vi "DAQWhichDevice.vi"(6 "error in":errorcluster caption="entrée d'erreur") -> (0 "error out":errorcluster caption="sortie d'erreur", 1 "AI.VoiesPhysiques":tag[](array[tag]), 2 "sourceTrig":tag, 3 "Message":string, 4 "DigitalInputFinAcq":tag, 5 "OK?":bool, 8 "Nom de périphérique DAQmx classique":tag)   [LabVIEW 2017]
uses:
  <resource>/objmgr/daqmx.rc
panel:
  out "AI.PhysicalChans":tag[](array[tag])
  out "error out 5":errorcluster
  out "résultat":i16
  out "0, 1":i16
  out "error out 4":errorcluster caption="sortie d'erreur"
  out "error out 3":errorcluster caption="sortie d'erreur"
  out "error out 2":errorcluster caption="sortie d'erreur"
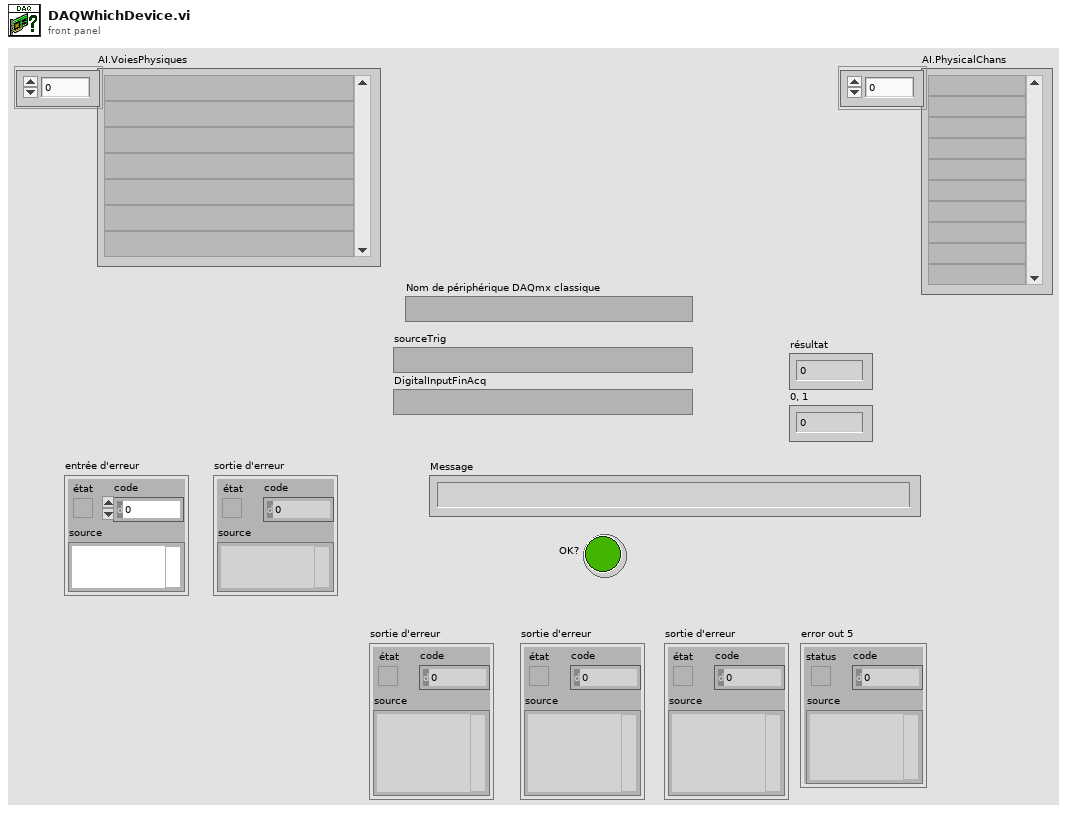
[diagram p1: front panel]
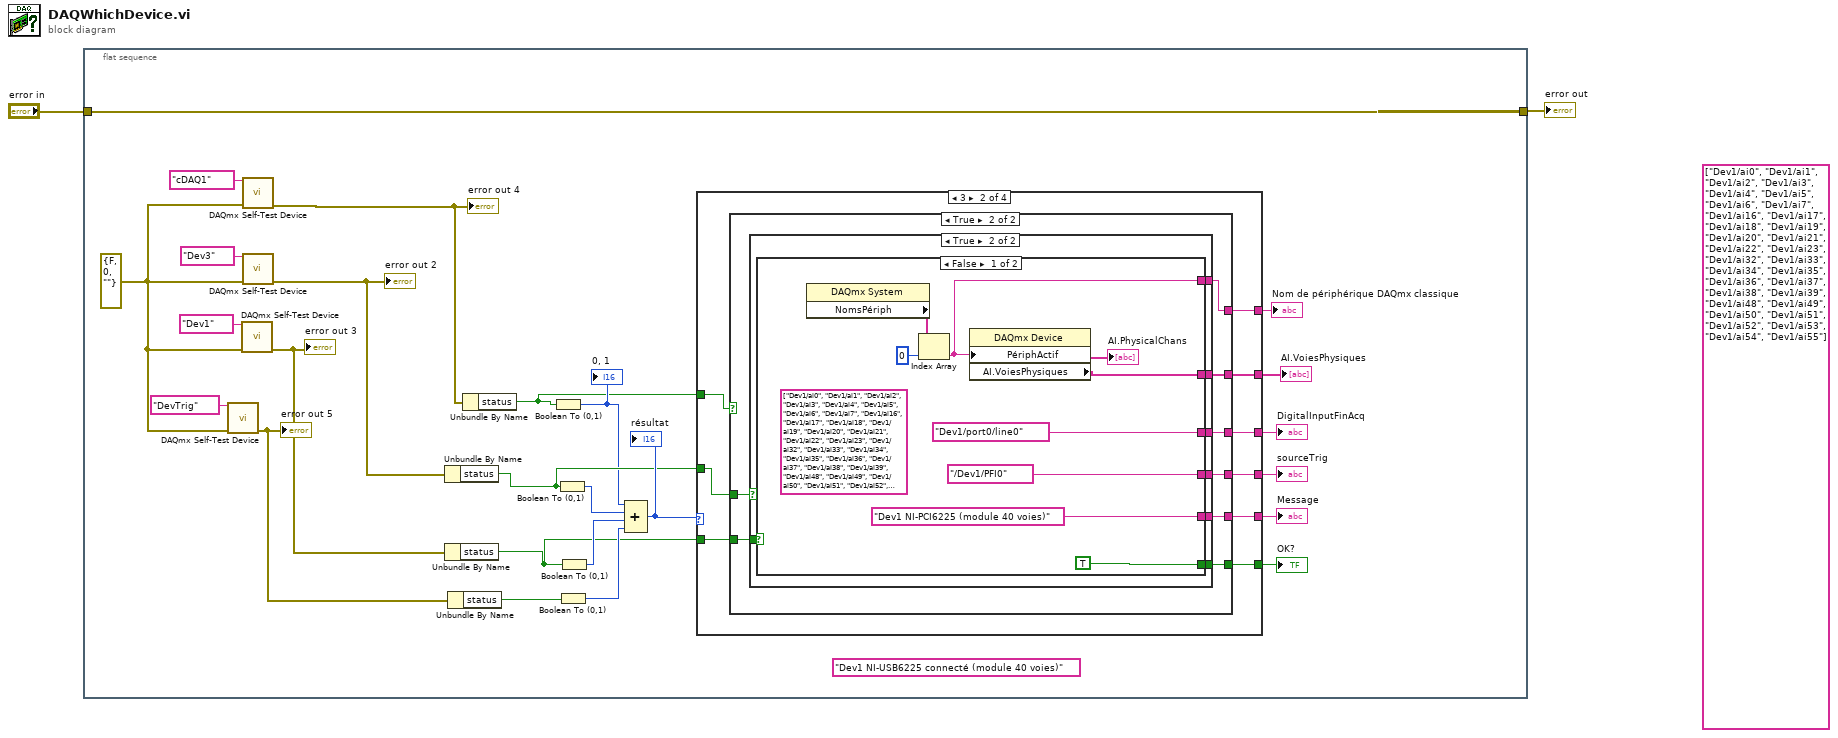
[diagram p0: block diagram]
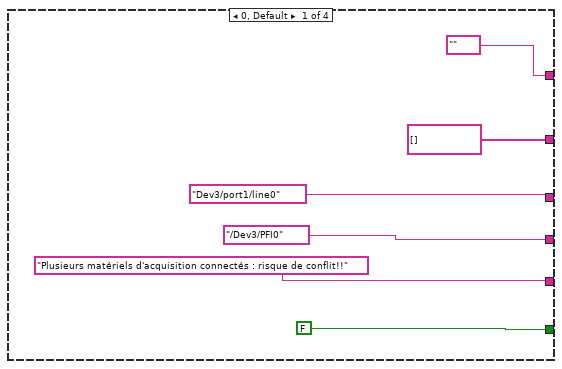
[diagram p2: hidden frame]
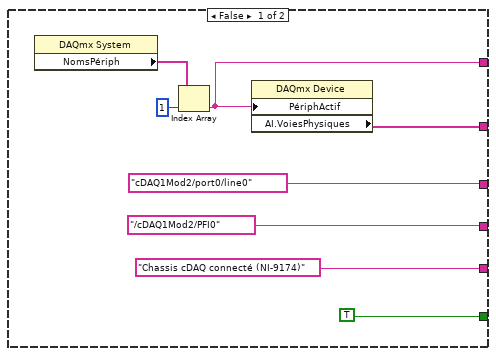
[diagram p3: hidden frame]
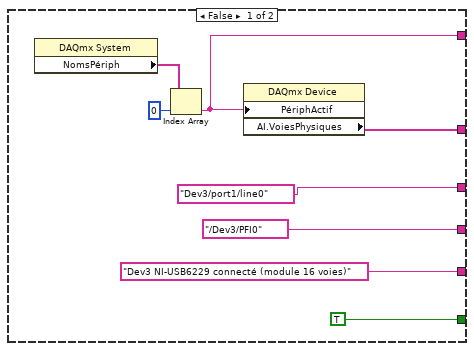
[diagram p4: hidden frame]
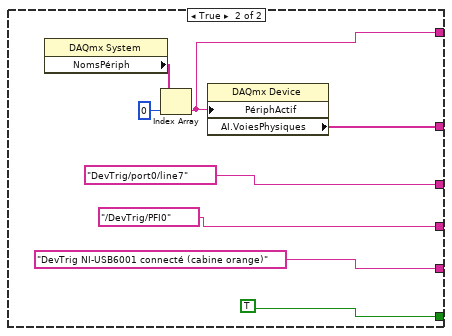
[diagram p5: hidden frame]
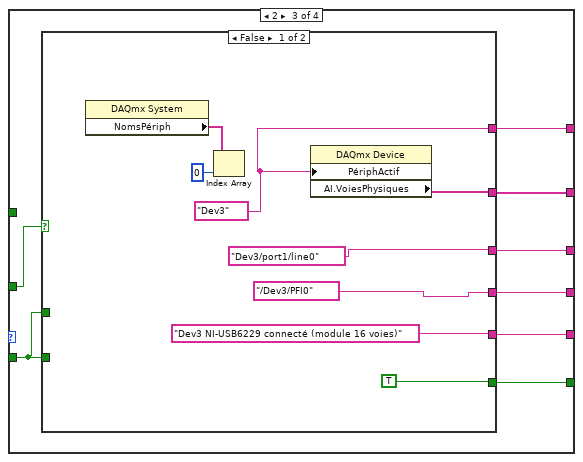
[diagram p6: hidden frame]
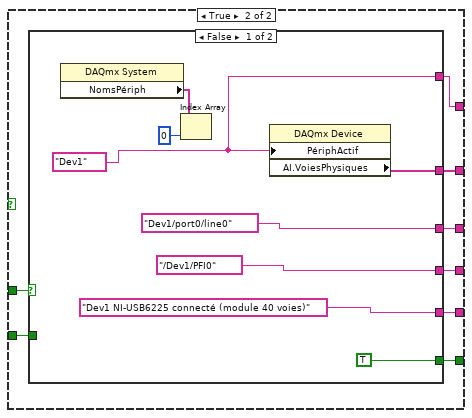
[diagram p7: hidden frame]
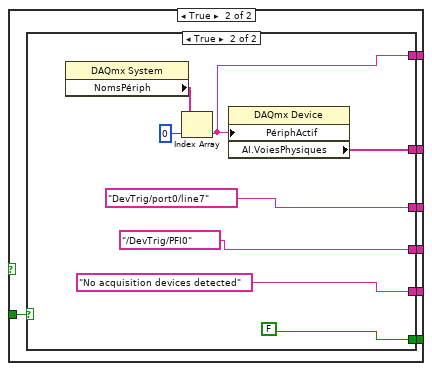
[diagram p8: hidden frame]
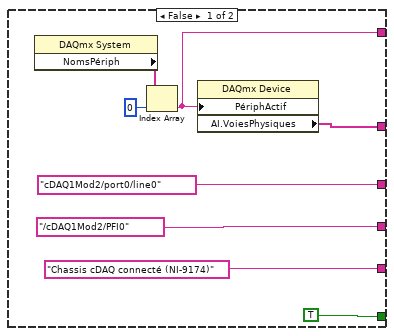
[diagram p9: hidden frame]
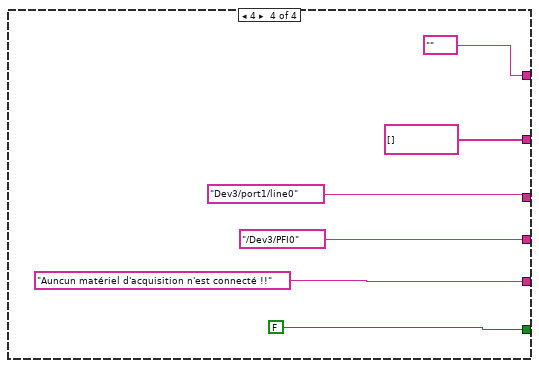
[diagram p10: hidden frame]
diagram:
  (unwired) tag[] ["Dev1/ai0", "Dev1/ai1", "Dev1/ai2", "Dev1/ai3", "Dev1/ai4", "Dev1/ai5", "Dev1/ai6", "Dev1/ai7", "Dev1/ai16", "Dev1/ai17", "Dev1/ai18", "Dev1/ai19", "Dev1/ai20", "Dev1/ai21", "Dev1/ai22", "Dev1/ai23", "Dev1/ai32", "Dev1/ai33", "Dev1/ai34", "Dev1/ai35", "Dev1/ai36", "Dev1/ai37", "Dev1/ai38", "Dev1/ai39", "Dev1/ai48", "Dev1/ai49", "Dev1/ai50", "Dev1/ai51", "Dev1/ai52", "Dev1/ai53", "Dev1/ai54", "Dev1/ai55"] ("AI.VoiesPhysiques 2")
  n1 = flat-sequence {
    tunnel: "error in" -> [w15]
    tunnel: [w15] -> w1
    frame #0 {
      (unwired) "Dev1 NI-USB6225 connecté (module 40 voies)"
      w7 = errorcluster {"status"=FALSE, "code"=0, "source"=""} ("error in")
      n2 = call <vilib>:"DAQmx Self-Test Device.vi"("device in"=tag "DevTrig", "error in"=w7) -> ("error out"=w5:errorcluster)  [unwired: 13 in]
      "error out 5" <- w5
      n3 = call <vilib>:"DAQmx Self-Test Device.vi"("device in"=tag "Dev1", "error in"=w7) -> ("error out"=w24:errorcluster)  [unwired: 13 in]
      "error out 3" <- w24
      n4 = call <vilib>:"DAQmx Self-Test Device.vi"("device in"=tag "cDAQ1", "error in"=w7) -> ("error out"=w13:errorcluster)  [unwired: 13 in]
      "error out 4" <- w13
      n5 = call <vilib>:"DAQmx Self-Test Device.vi"("device in"=tag "Dev3", "error in"=w7) -> ("error out"=w25:errorcluster)  [unwired: 13 in]
      "error out 2" <- w25
      n6 = Unbundle By Name(w25) -> ("status"=w17:bool)
      n7 = Unbundle By Name(w24) -> ("status"=w3:bool)
      n8 = Unbundle By Name(w5) -> ("status"=w6:bool)
      n9 = Unbundle By Name(w13) -> ("status"=w11:bool)
      n10 = Boolean To (0,1)(Boolean=w11) -> (0, 1=w12:i16)
      "0, 1" <- w12
      n11 = Boolean To (0,1)(Boolean=w17) -> (0, 1=w23:i16)
      n12 = Boolean To (0,1)(Boolean=w6) -> (0, 1=w4:i16)
      n13 = Boolean To (0,1)(Boolean=w3) -> (0, 1=w22:i16)
      n14 = Compound Arithmetic op=ADD(w12, w23, w22, w4) -> (w21:i16)
      "résultat" <- w21
      n15 = case shown="3" w21 {
        tunnel: ["Plusieurs matériels d'acquisition connectés : risque de conflit!!" w41 w97 "Auncun matériel d'acquisition n'est connecté !!"] -> w20
        tunnel: w17 -> [_ w42 w91 _]
        tunnel: [FALSE ("OK?") w40 w96 FALSE ("OK?")] -> w19
        tunnel: [tag "/Dev3/PFI0" ("source") w39 w95 tag "/Dev3/PFI0" ("source")] -> w18
        tunnel: [tag "Dev3/port1/line0" ("lines") w38 w94 tag "Dev3/port1/line0" ("lines")] -> w16
        tunnel: w11 -> [_ w37 _ _]
        tunnel: [tag[] [] ("AI.VoiesPhysiques") w36 w93 tag[] [] ("AI.VoiesPhysiques")] -> w10
        tunnel: [tag "" w35 w92 tag ""] -> w9
        tunnel: w3 -> [_ w34 w90 _]
        frame 0, Default {
        }
        frame 3 {
          n16 = case shown="True" w37 {
            tunnel: w42 -> [_ w58]
            tunnel: ["Chassis cDAQ connecté (NI-9174)" w57] -> w41
            tunnel: [TRUE ("OK?") w56] -> w40
            tunnel: [tag "/cDAQ1Mod2/PFI0" ("source") w55] -> w39
            tunnel: [tag "cDAQ1Mod2/port0/line0" ("lines") w54] -> w38
            tunnel: [w44 w53] -> w36
            tunnel: [w43 w52] -> w35
            tunnel: w34 -> [_ w51]
            frame False {
              n17 = property class="DAQmx System"() -> ("NomsPériph"=w45:tag[])  [unwired: 2 in, 2 out]
              n18 = Index Array(array=w45, index=1 ("indice")) -> (element=w43:tag)
              n19 = property class="DAQmx Device"("PériphActif"=w43) -> ("AI.VoiesPhysiques"=w44:tag[])  [unwired: 2 in, 2 out]
            }
            frame True {
              n20 = case shown="True" w58 {
                tunnel: ["Dev3 NI-USB6229 connecté (module 16 voies)" w73] -> w57
                tunnel: [TRUE ("OK?") w72] -> w56
                tunnel: [tag "/Dev3/PFI0" ("source") w71] -> w55
                tunnel: [tag "Dev3/port1/line0" ("lines") w70] -> w54
                tunnel: [w60 w67] -> w53
                tunnel: [w59 w69] -> w52
                tunnel: w51 -> [_ w68]
                frame False {
                  n21 = property class="DAQmx System"() -> ("NomsPériph"=w62:tag[])  [unwired: 2 in, 2 out]
                  n22 = Index Array(array=w62, index=0 ("indice")) -> (element=w59:tag)
                  n23 = property class="DAQmx Device"("PériphActif"=w59) -> ("AI.VoiesPhysiques"=w60:tag[])  [unwired: 2 in, 2 out]
                }
                frame True {
                  n24 = case shown="False" w68 {
                    tunnel: ["Dev1 NI-PCI6225 (module 40 voies)" "DevTrig NI-USB6001 connecté (cabine orange)"] -> w73
                    tunnel: [TRUE ("OK?") TRUE ("OK?")] -> w72
                    tunnel: [tag "/Dev1/PFI0" ("source") tag "/DevTrig/PFI0" ("source")] -> w71
                    tunnel: [tag "Dev1/port0/line0" ("lines") tag "DevTrig/port0/line7" ("lines")] -> w70
                    tunnel: [w74 w82] -> w67
                    tunnel: [w75 w87] -> w69
                    frame False {
                      (unwired) tag[] ["Dev1/ai0", "Dev1/ai1", "Dev1/ai2", "Dev1/ai3", "Dev1/ai4", "Dev1/ai5", "Dev1/ai6", "Dev1/ai7", "Dev1/ai16", "Dev1/ai17", "Dev1/ai18", "Dev1/ai19", "Dev1/ai20", "Dev1/ai21", "Dev1/ai22", "Dev1/ai23", "Dev1/ai32", "Dev1/ai33", "Dev1/ai34", "Dev1/ai35", "Dev1/ai36", "Dev1/ai37", "Dev1/ai38", "Dev1/ai39", "Dev1/ai48", "Dev1/ai49", "Dev1/ai50", "Dev1/ai51", "Dev1/ai52", "Dev1/ai53", "Dev1/ai54", "Dev1/ai55"] ("AI.VoiesPhysiques 2")
                      n25 = property class="DAQmx System"() -> ("NomsPériph"=w77:tag[])  [unwired: 2 in, 2 out]
                      n26 = Index Array(array=w77, index=0 ("indice")) -> (element=w75:tag)
                      n27 = property class="DAQmx Device"("PériphActif"=w75) -> ("AI.VoiesPhysiques"=w74:tag[])  [unwired: 2 in, 2 out]
                      "AI.PhysicalChans" <- w74
                    }
                    frame True {
                      n28 = property class="DAQmx System"() -> ("NomsPériph"=w89:tag[])  [unwired: 2 in, 2 out]
                      n29 = Index Array(array=w89, index=0 ("indice")) -> (element=w87:tag)
                      n30 = property class="DAQmx Device"("PériphActif"=w87) -> ("AI.VoiesPhysiques"=w82:tag[])  [unwired: 2 in, 2 out]
                    }
                  }
                }
              }
            }
          }
        }
        frame 2 {
          n31 = case shown="False" w91 {
            tunnel: w90 -> [_ w113]
            tunnel: ["Dev3 NI-USB6229 connecté (module 16 voies)" w112] -> w97
            tunnel: [TRUE ("OK?") w111] -> w96
            tunnel: [tag "/Dev3/PFI0" ("source") w110] -> w95
            tunnel: [tag "Dev3/port1/line0" ("lines") w109] -> w94
            tunnel: [w99 w108] -> w93
            tunnel: [w98 w107] -> w92
            tunnel: w90 -> [_ w106]
            frame False {
              w98 = tag "Dev3" ("device in")
              n32 = property class="DAQmx System"() -> ("NomsPériph"=w105:tag[])  [unwired: 2 in, 2 out]
              n33 = Index Array(array=w105, index=0 ("indice")) -> ()  [unwired: 1 out]
              n34 = property class="DAQmx Device"("PériphActif"=w98) -> ("AI.VoiesPhysiques"=w99:tag[])  [unwired: 2 in, 2 out]
            }
            frame True {
              n35 = case shown="False" w113 {
                tunnel: ["Dev1 NI-USB6225 connecté (module 40 voies)" w128] -> w112
                tunnel: [TRUE ("OK?") w127] -> w111
                tunnel: [tag "/Dev1/PFI0" ("source") w126] -> w110
                tunnel: [tag "Dev1/port0/line0" ("lines") w125] -> w109
                tunnel: [w118 w124] -> w108
                tunnel: [w114 w123] -> w107
                tunnel: w106 -> [_ w122]
                frame False {
                  w114 = tag "Dev1" ("Nom de périphérique DAQmx classique 2")
                  n36 = property class="DAQmx System"() -> ("NomsPériph"=w120:tag[])  [unwired: 2 in, 2 out]
                  n37 = Index Array(array=w120, index=0 ("indice")) -> ()  [unwired: 1 out]
                  n38 = property class="DAQmx Device"("PériphActif"=w114) -> ("AI.VoiesPhysiques"=w118:tag[])  [unwired: 2 in, 2 out]
                }
                frame True {
                  n39 = case shown="True" w122 {
                    tunnel: ["Chassis cDAQ connecté (NI-9174)" "No acquisition devices detected"] -> w128
                    tunnel: [TRUE ("OK?") FALSE ("OK?")] -> w127
                    tunnel: [tag "/cDAQ1Mod2/PFI0" ("source") tag "/DevTrig/PFI0" ("source")] -> w126
                    tunnel: [tag "cDAQ1Mod2/port0/line0" ("lines") tag "DevTrig/port0/line7" ("lines")] -> w125
                    tunnel: [w133 w142] -> w124
                    tunnel: [w132 w141] -> w123
                    frame False {
                      n40 = property class="DAQmx System"() -> ("NomsPériph"=w135:tag[])  [unwired: 2 in, 2 out]
                      n41 = Index Array(array=w135, index=0 ("indice")) -> (element=w132:tag)
                      n42 = property class="DAQmx Device"("PériphActif"=w132) -> ("AI.VoiesPhysiques"=w133:tag[])  [unwired: 2 in, 2 out]
                    }
                    frame True {
                      n43 = property class="DAQmx System"() -> ("NomsPériph"=w144:tag[])  [unwired: 2 in, 2 out]
                      n44 = Index Array(array=w144, index=0 ("indice")) -> (element=w141:tag)
                      n45 = property class="DAQmx Device"("PériphActif"=w141) -> ("AI.VoiesPhysiques"=w142:tag[])  [unwired: 2 in, 2 out]
                    }
                  }
                }
              }
            }
          }
        }
        frame 4 {
        }
      }
      "Message" <- w20
      "OK?" <- w19
      "sourceTrig" <- w18
      "DigitalInputFinAcq" <- w16
      "AI.VoiesPhysiques" <- w10
      "Nom de périphérique DAQmx classique" <- w9
    }
  }
  "error out" <- w1
